vi "Multiple AOIs.vi"(4 "White level":dbl=255.0 format="%.2f", 5 "Black level":dbl format="%.2f", 6 "First (or only) image (red)":T2, 8 "error in":errorcluster, 9 "Second image (green)":T2, 11 "Image Type":u32(ring) items=["8 bits", "16 bits", "Float", "Complex", "RGB", "HSL"]) -> (0 "error out":errorcluster)   [LabVIEW 2011]
doc: "Use to designate multiple areas of interest (AOIs) in the image"
uses:
  <vilib>/vision/Image Controls.llb/IMAQ Image.ctl
  AOI List Globals.vi
  <vilib>/vision/NI_Vision_Development_Module.lvlib
  <vilib>/Utility/NIReport.llb/NI_ReportGenerationCore.lvlib
  <vilib>/Analysis/NI_AALBase.lvlib
panel:
  in  "Case Constant\n(See Context Help)":bool
  in  "Printer":u16(ring) items=["QBIO lab Lexmark C532 PS3", "Microsoft XPS Document Writer", "Microsoft Office Document Image Writer", "Lab Zippy  (jg-zippy.kosow.brandeis.edu)", "Lab hp color LaserJet 2550 PS", "Journal Note Writer", "HP Universal Printing PS", "HP Universal Printing PCL 6", "Home HP LaserJet 4L", "Fax", "Adobe PDF", "\\\\BASEMENT\\Home EPSON Stylus Photo 1400 Series", "\\\\jg-x\\Jeff's office EPSON Stylus CX7400 Series 2"]
  in  "Print AOIs":bool
  in  "Resize all AOIs":bool
  in  "Read AOI list from file":bool
  in  "Save AOI list to file":bool
  in  "Y":u16(slide)=20 caption="Fixed AOI Y size" max=480 scale=0.0..50.0
  in  "X":u16(slide)=20 caption="Fixed AOI X size" max=640 scale=0.0..50.0
  in  "Delete all AOIs":bool
  in  "Mouse Operation to perform":T1(ring)
  in  "Exit":bool
  # "Ordinarily not for interactive use:"
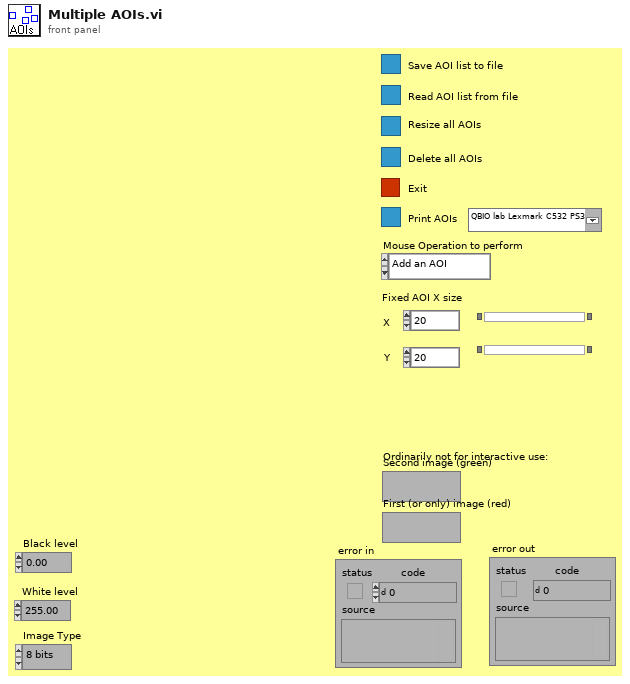
[diagram p1: front panel]
types:
  T1 = enum16{"Add an AOI", "Resize an AOI", "Delete an AOI"}
  T2 = typedef "IMAQ Image.ctl" = refnum<image>
  T3 = enum32{"8 bits", "16 bits", "Float", "Complex", "RGB Chunky", "Compressed"}
  T4 = enum32{"No Selection", "Point", "Line", "Rectangle", "Oval", "Polygon", "Free", "Unused1", "Zoom", "Unused2", "Broken Line", "Free Hand Line"}
  T5 = enum32{"No Selection", "Point", "Line", "Rectangle", "Oval", "Polygon", "Free", "Unused1", "Zoom", "Unused2", "Broken Line", "Free Hand Line"}[]
  T6 = enum32{"No  event", "Click event", "Draw event", "Move event", "Size event", "Scroll event", "Activate event", "Close event", "Reserved"}[]
  T7 = cluster{"AOI List[0]":u16, "AOI List[1]":u16, "AOI List[2]":u16, "AOI List[3]":u16}
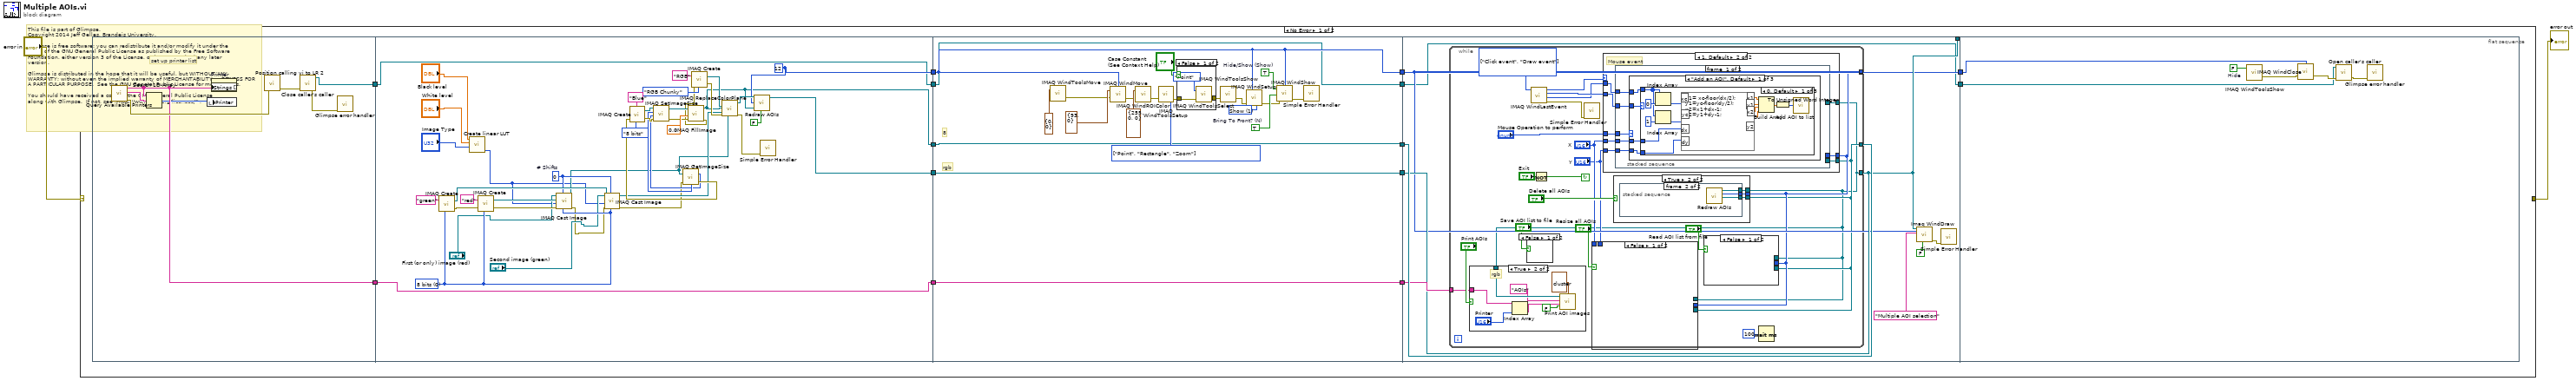
[diagram p0: block diagram]
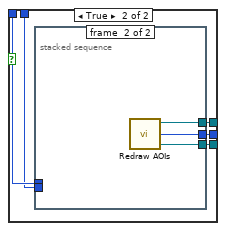
[diagram p4: hidden frame]
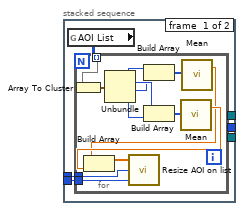
[diagram p5: hidden frame]
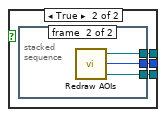
[diagram p6: hidden frame]
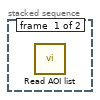
[diagram p7: hidden frame]
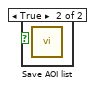
[diagram p8: hidden frame]
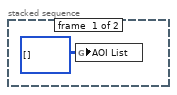
[diagram p10: hidden frame]
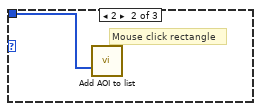
[diagram p12: hidden frame]
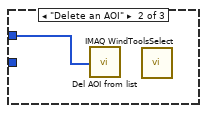
[diagram p14: hidden frame]
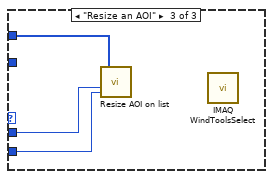
[diagram p15: hidden frame]
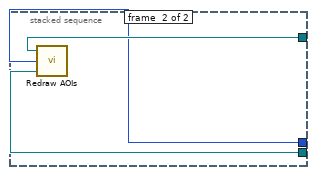
[diagram p16: hidden frame]
diagram:
  # "This file is part of Glimpse. \nCopyright 2014 Jeff Gelles, Brandeis University.    \n\nGlimpse is free software: you can redistribute it and/or modify it under the \nterms of the GNU General Public License as published by the Free Software \nFoundation, either version 3 of the License, or (at your option) any later \nversion.\n\nGlimpse is distributed in the hope that it will be useful, but WITHOUT ANY \nWARRANTY; without even the implied warranty of MERCHANTABILITY or FITNESS FOR \nA PARTICULAR PURPOSE.  See the GNU General Public License for more details.\n\nYou should have received a copy of the GNU General Public License\nalong with Glimpse.  If not, see <http://www.gnu.org/licenses/>."
  n1 = case shown="No Error" "error in" {
    selector: "error in" -> [_ w206]
    tunnel: [_ w206] -> w1
    frame No Error {
      n2 = flat-sequence {
        tunnel: [w22] -> w16
        tunnel: [w19] -> w15
        tunnel: [w50] -> w14
        tunnel: [w52] -> w13
        tunnel: [w38] -> w12
        tunnel: w16 -> [w25]
        tunnel: [w25] -> w11
        tunnel: w15 -> [w24]
        tunnel: [w24] -> w10
        tunnel: w14 -> [w69]
        tunnel: [w69] -> w9
        tunnel: w13 -> [w68]
        tunnel: [w68] -> w8
        tunnel: w12 -> [w67]
        tunnel: [w67] -> w7
        tunnel: w11 -> [w66]
        tunnel: [w66] -> w6
        tunnel: w10 -> [w65]
        tunnel: [w65] -> w5
        tunnel: [w95] -> _
        tunnel: w9 -> [w91]
        tunnel: [w91] -> w4
        tunnel: w8 -> [w95]
        tunnel: w7 -> [w97]
        tunnel: w6 -> [w90]
        tunnel: [w90] -> w3
        tunnel: w5 -> [w96]
        tunnel: w4 -> [w204]
        tunnel: w3 -> [w200]
        frame #0 {
          # "set up printer list"
          n3 = call <vilib>:"Query Available Printers.vi"() -> ("error out"=w20:errorcluster, "default printer"=w18:string, "system configured printers"=w19:string[])  [unwired: 1 in, 8 out]
          n4 = Search 1D Array(1D array=w19, element=w18) -> (index of element=w17:i32)  [unwired: 1 out]
          n5 = local write "Printer"(w17) -> ()
          n6 = property on="Printer" class="Ring (strict)"("Strings []"=w19) -> ()  [unwired: 2 in, 2 out]
          n7 = call "Position calling vi to LR 2.vi"("error in (no error)"=w20) -> ("error out"=w23:errorcluster)  [unwired: 1 in, 3 out]
          n8 = call "Close caller's caller.vi"("error in (no error)"=w23) -> ("error out"=w21:errorcluster, "vi reference"=w22:refnum<vi>)  [unwired: 6 out]
          n9 = call "Glimpse error handler.vi"("error in"=w21) -> ()  [unwired: 1 in, 6 out]
        }
        frame #1 {
          w39 = 0  # # Shifts
          w44 = u32 0 items=["8 bits", "16 bits", "Float", "Complex", "RGB", "HSL"] ("Image Type")
          w50 = 12 ("Window Number (0...15)")
          n10 = call "IMAQ Create"("Image Name"="green", "Image Type"=w44) -> ("New Image"=w42:T2, "error out"=w45:errorcluster)  [unwired: 2 in, 1 out]
          n11 = call "Create linear LUT.vi"("Input Image Type"="Image Type", "White Value"="White level", "Black Value"="Black level") -> ("LUT (U8) Out"=w28:u8[])  [unwired: 1 in, 5 out]
          n12 = call "IMAQ Create"("Image Name"="red", "Image Type"=w44, "error in (no error)"=w45) -> ("New Image"=w43:T2, "error out"=w31:errorcluster)  [unwired: 1 in, 1 out]
          n13 = call "IMAQ Cast Image"("Image Type"=w44, "# Shifts"=w39, "error in (no error)"=w31, "Lookup Table"=w28, "Image Dst"=w43, "Image Src"="First (or only) image (red)") -> ("error out"=w27:errorcluster, "Image Dst Out"=w37:T2)  [unwired: 4 out]
          n14 = call "IMAQ Cast Image"("Image Type"=w44, "# Shifts"=w39, "error in (no error)"=w27, "Lookup Table"=w28, "Image Dst"=w42, "Image Src"="Second image (green)") -> ("error out"=w46:errorcluster, "Image Dst Out"=w47:T2)  [unwired: 4 out]
          n15 = call "IMAQ GetImageSize"("Image"=w37, "error in (no error)"=w46) -> ("Y Resolution"=w48:i32, "X Resolution"=w49:i32, "error out"=w53:errorcluster)  [unwired: 2 out]
          n16 = call "IMAQ Create"("Image Name"="Blue", "Image Type"=T3."8 bits", "error in (no error)"=w53) -> ("New Image"=w57:T2, "error out"=w56:errorcluster)  [unwired: 1 in, 1 out]
          n17 = call "IMAQ SetImageSize"("error in (no error)"=w56, "Y Resolution"=w48, "X Resolution"=w49, "Image"=w57) -> ("error out"=w54:errorcluster, "Image Out"=w55:T2)  [unwired: 1 out]
          n18 = call "IMAQ FillImage"("error in (no error)"=w54, "Pixel Value (U8, U16, I16, Float)"=sgl 0.0 ("Pixel Value (U8, I16, Float)"), "Image"=w55) -> ("error out"=w33:errorcluster, "Image Out"=w38:T2)  [unwired: 4 in, 3 out]
          n19 = call "IMAQ Create"("Image Name"="RGB", "Image Type"=T3."RGB Chunky", "error in (no error)"=w33) -> ("New Image"=w62:T2, "error out"=w61:errorcluster)  [unwired: 1 in, 1 out]
          n20 = call "IMAQ ReplaceColorPlane"("Image Dst"=w62, "Red or Hue Plane"=w38, "Green or Sat Plane"=w47, "error in (no error)"=w61, "Blue or Luma or Val or Inten Plane"=w37) -> ("Image Dst Out"=w51:T2, "error out"=w32:errorcluster)  [unwired: 2 in, 7 out]
          n21 = call "Redraw AOIs.vi"("Resize to Image Size?"=FALSE, "Image Src (Red Plane)"=w38, "Window Number (0...15)"=w50, "Image Src (RGB)"=w51) -> ("Image Dst Out (RGB)"=w52:T2)  [unwired: 1 out]
          n22 = call <vilib>:"Simple Error Handler.vi"("error in (no error)"=w32) -> ()  [unwired: 1 in, 8 out]
        }
        frame #2 {
          w70 = 1 items=["Hide", "Show", "No change"] ("Scrollbars (No change)")
          w77 = TRUE  # Bring To Front? (N)
          w78 = TRUE  # Hide/Show (Show)
          w83 = T5 [enum."Point", enum."Rectangle", enum."Zoom"] items=["No Selection", "Point", "Line", "Rectangle", "Oval", "Polygon", "Free", "Unused1", "Zoom", "Unused2", "Broken Line", "Free Hand Line"] ("Tools")
          # "rgb"
          # "8"
          n23 = call "IMAQ WindToolsMove"("Coordinates"=cluster{"X Position":i32, "Y Position":i32} {"X Position"=0, "Y Position"=0}) -> ("error out"=w73:errorcluster)  [unwired: 2 in, 3 out]
          n24 = call "IMAQ WindMove"("Window Number (0...15)"=w69, "Coordinates (screen)"=cluster{"X Position":i32, "Y Position":i32} {"X Position"=93, "Y Position"=0}, "error in (no error)"=w73) -> ("error out"=w72:errorcluster)  [unwired: 1 in, 2 out]
          n25 = call "IMAQ WindROIColor"("Color of ROI (white)"=cluster{"Red":u8, "Green":u8, "Blue":u8} {"Red"=255, "Green"=0, "Blue"=0}, "error in (no error)"=w72) -> ("error out"=w84:errorcluster)  [unwired: 4 out]
          n26 = call "IMAQ WindToolsSetup"("Tools"=w83, "error in (no error)"=w84) -> ("error out"=w82:errorcluster)  [unwired: 2 in, 2 out]
          n27 = case shown="False" "Case Constant\n(See Context Help)" {
            tunnel: w82 -> [w87 w89]
            tunnel: [w86 w89] -> w81
            frame False {
              n28 = call "IMAQ WindToolsSelect"("Tool (Point)"=T4."Point", "error in (no error)"=w87) -> ("error out"=w86:errorcluster)  [unwired: 2 in, 2 out]
            }
            frame True {
            }
          }
          n29 = call "IMAQ WindToolsShow"("error in (no error)"=w81) -> ("error out"=w80:errorcluster)  [unwired: 2 in, 3 out]
          n30 = call "IMAQ WindSetup"("Scrollbars (No change)"=w70, "Window Number (0...15)"=w69, "error in (no error)"=w80) -> ("error out"=w71:errorcluster)  [unwired: 4 in, 4 out]
          n31 = call "IMAQ WindShow"("error in (no error)"=w71, "Bring To Front? (N)"=w77, "Hide/Show (Show)"=w78, "Window Number (0...15)"=w69) -> ("error out"=w79:errorcluster)  [unwired: 1 in, 3 out]
          n32 = call <vilib>:"Simple Error Handler.vi"("error in (no error)"=w79) -> ()  [unwired: 1 in, 8 out]
        }
        frame #3 {
          n33 = while {
            tunnel: w95 -> [w99]
            tunnel: w97 -> [w103]
            tunnel: w91 -> [w104]
            tunnel: w91 -> [_]
            tunnel: w96 -> [w98]
            stop <- w116 continue-if-true
            w115 = T6 [enum."Click event", enum."Draw event"] items=["No  event", "Click event", "Draw event", "Move event", "Size event", "Scroll event", "Activate event", "Close event", "Reserved"] ("Events list (all)")
            n34 = case shown="True" "Print AOIs" {
              tunnel: w99 -> [_ w124]
              tunnel: w98 -> [_ w121]
              frame False {
              }
              frame True {
                # "rgb"
                n35 = Index Array(array=w121, index="Printer") -> (element=w123:string)
                n36 = call "Print AOI images.vi"("Black/White Levels"=cluster{ext, ext} {0.0, 255.0}, "AOI Overlay?"=FALSE, "printer name (default)"=w123, "Printout title"="AOIs", "Image In"=w124) -> ()  [unwired: 1 in, 5 out]
              }
            }
            n37 = case shown="False" "Save AOI list to file" {
              frame False {
              }
              frame True {
                n38 = call "Save AOI list.vi"() -> ()  [unwired: 1 out]
              }
            }
            n39 = call "IMAQ WindLastEvent"("Events list (all)"=w115) -> ("error out"=w101:errorcluster, "Coordinates"=w111:i32[], "Tool"=w112:i32, "Event"=w114:i32)  [unwired: 1 in, 6 out]
            n40 = Not(x="Exit") -> (.not. x?=w116:bool)
            n41 = call <vilib>:"Simple Error Handler.vi"("error in (no error)"=w101) -> ()  [unwired: 1 in, 8 out]
            n42 = case shown="False" "Resize all AOIs" {
              tunnel: "X" -> [_ w129]
              tunnel: "Y" -> [_ w128]
              tunnel: w99 -> [_ w127]
              tunnel: w104 -> [_ w126]
              tunnel: w103 -> [_ w125]
              frame False {
              }
              frame True {
                n43 = stacked-sequence {
                  tunnel: w129 -> [w132 _]
                  tunnel: w128 -> [w131 _]
                  tunnel: w127 -> [_ w148]
                  tunnel: w126 -> [_ w147]
                  tunnel: w125 -> [_ w146]
                  frame #0 {
                    n44 = global read "AOI List Globals.vi" "AOI List"() -> (w130:u16[][])
                    n45 = for {
                      tunnel: w132 -> [w145]
                      tunnel: w131 -> [w144]
                      tunnel: w130 -> [w142] mode=indexing
                      n46 = Array To Cluster(array=w142) -> (cluster=w141:T7)
                      n47 = Unbundle(w141) -> ("AOI List[0]"=w140:u16, "AOI List[1]"=w139:u16, "AOI List[2]"=w138:u16, "AOI List[3]"=w137:u16)
                      n48 = Build Array(w140, w138) -> (w136:u16[])
                      n49 = Build Array(w139, w137) -> (w135:u16[])
                      n50 = call <vilib>:"Mean.vi"("X"=w135) -> ("mean"=w134:dbl)  [unwired: 1 out]
                      n51 = call <vilib>:"Mean.vi"("X"=w136) -> ("mean"=w133:dbl)  [unwired: 1 out]
                      n52 = Build Array(w133, w134) -> (w143:dbl[])
                      n53 = call "Resize AOI on list.vi"("New y dimension"=w144, "New x dimension"=w145, "Coordinates of  AOI to resize"=w143) -> ()  [unwired: 2 out]
                    }
                  }
                  frame #1 {
                    n54 = call "Redraw AOIs.vi"("Image Src (Red Plane)"=w146, "Window Number (0...15)"=w147, "Image Src (RGB)"=w148) -> ()  [unwired: 1 in, 2 out]
                  }
                }
              }
            }
            n55 = case shown="1, Default" w114 {
              tunnel: "Mouse Operation to perform" -> [_ w169]
              tunnel: w112 -> [_ w168]
              tunnel: w111 -> [_ w167]
              tunnel: w104 -> [_ w166]
              tunnel: w103 -> [_ w165]
              tunnel: w99 -> [_ w164]
              tunnel: "X" -> [_ w163]
              tunnel: "Y" -> [_ w162]
              frame 0 {
                # "No mouse event"
              }
              frame 1, Default {
                # "Mouse event"
                n56 = stacked-sequence {
                  tunnel: w169 -> [w174 _]
                  tunnel: w168 -> [w173 _]
                  tunnel: w167 -> [w172 _]
                  tunnel: w166 -> [_ w198]
                  tunnel: w165 -> [_ w197]
                  tunnel: w164 -> [_ w199]
                  tunnel: w163 -> [w171 _]
                  tunnel: w162 -> [w170 _]
                  frame #0 {
                    n57 = case shown="\"Add an AOI\", Default" w174 {
                      tunnel: w173 -> [w178 _ _]
                      tunnel: w172 -> [w177 w193 w194]
                      tunnel: w171 -> [w176 _ w196]
                      tunnel: w170 -> [w175 _ w195]
                      frame "Add an AOI", Default {
                        n58 = case shown="0, Default" w178 {
                          tunnel: w177 -> [w189 w192 _]
                          tunnel: w176 -> [w182 _ _]
                          tunnel: w175 -> [w181 _ _]
                          frame 0, Default {
                            # "Mouse click point"
                            n59 = Index Array(array=w189, index=0) -> (element=w188:i32)
                            n60 = Index Array(array=w189, index=1) -> (element=w187:i32)
                            n61 = formula code="x1= xc-floor(dx/2);\ny1=yc-floor(dy/2);\nx2=x1+dx-1;\ny2=y1+dy-1;"("xc"=w188, "yc"=w187, "dx"=w182, "dy"=w181) -> ("x1"=w185:dbl, "y1"=w186:dbl, "x2"=w184:dbl, "y2"=w183:dbl)
                            n62 = Build Array(w185, w186, w184, w183) -> (w179:dbl[])
                            n63 = To Unsigned Word Integer(number=w179) -> (unsigned 16bit integer=w180:u16[])
                            n64 = call "Add AOI to list.vi"("AOI to add"=w180) -> ()  [unwired: 1 out]
                          }
                          frame 2 {
                            # "Mouse click rectangle"
                            n65 = call "Add AOI to list.vi"("AOI to add"=w192) -> ()  [unwired: 1 out]
                          }
                          frame 8 {
                            # "zoom -- no action"
                          }
                        }
                      }
                      frame "Delete an AOI" {
                        n66 = call "Del AOI from list.vi"("Coordinates of  AOI to delete"=w193) -> ()  [unwired: 1 out]
                        n67 = call "IMAQ WindToolsSelect"() -> ()  [unwired: 4 in, 3 out]
                      }
                      frame "Resize an AOI" {
                        n68 = call "Resize AOI on list.vi"("New y dimension"=w195, "New x dimension"=w196, "Coordinates of  AOI to resize"=w194) -> ()  [unwired: 2 out]
                        n69 = call "IMAQ WindToolsSelect"() -> ()  [unwired: 4 in, 3 out]
                      }
                    }
                  }
                  frame #1 {
                    n70 = call "Redraw AOIs.vi"("Image Src (Red Plane)"=w197, "Window Number (0...15)"=w198, "Image Src (RGB)"=w199) -> ()  [unwired: 1 in, 2 out]
                  }
                }
              }
            }
            n71 = case shown="True" "Delete all AOIs" {
              tunnel: w104 -> [_ w157]
              tunnel: w103 -> [_ w156]
              tunnel: w99 -> [_ w155]
              frame False {
              }
              frame True {
                n72 = stacked-sequence {
                  tunnel: w157 -> [_ w160]
                  tunnel: w156 -> [_ w159]
                  tunnel: w155 -> [_ w161]
                  frame #0 {
                    n73 = global write "AOI List Globals.vi" "AOI List"(i32[][] []) -> ()
                  }
                  frame #1 {
                    n74 = call "Redraw AOIs.vi"("Image Src (Red Plane)"=w159, "Window Number (0...15)"=w160, "Image Src (RGB)"=w161) -> ()  [unwired: 1 in, 2 out]
                  }
                }
              }
            }
            n75 = case shown="False" "Read AOI list from file" {
              tunnel: w99 -> [_ w151]
              tunnel: w104 -> [_ w150]
              tunnel: w103 -> [_ w149]
              frame False {
              }
              frame True {
                n76 = stacked-sequence {
                  tunnel: w151 -> [_ w154]
                  tunnel: w150 -> [_ w153]
                  tunnel: w149 -> [_ w152]
                  frame #0 {
                    n77 = call "Read AOI list.vi"() -> ()  [unwired: 2 out]
                  }
                  frame #1 {
                    n78 = call "Redraw AOIs.vi"("Image Src (Red Plane)"=w152, "Window Number (0...15)"=w153, "Image Src (RGB)"=w154) -> ()  [unwired: 1 in, 2 out]
                  }
                }
              }
            }
            n79 = Wait (ms)(milliseconds to wait=u32 100) -> ()  [unwired: 1 out]
          }
          n80 = call "Imaq WindDraw"("Resize to Image Size? (Y)"=FALSE, "Window Number (0...15)"=w91, "Title"="Multiple AOI selection", "Image"=w95) -> ("error out"=w93:errorcluster)  [unwired: 2 in, 5 out]
          n81 = call <vilib>:"Simple Error Handler.vi"("error in (no error)"=w93) -> ()  [unwired: 1 in, 8 out]
        }
        frame #4 {
          w205 = FALSE  # Hide
          n82 = call "IMAQ WindToolsShow"("Hide/Show (Show)"=w205) -> ("error out"=w203:errorcluster)  [unwired: 2 in, 3 out]
          n83 = call "IMAQ WindClose"("Window Number (0...15)"=w204, "error in (no error)"=w203) -> ("error out"=w202:errorcluster)  [unwired: 1 in, 3 out]
          n84 = call "Open caller's caller.vi"("error in (no error)"=w202, "vi reference"=w200) -> ("error out"=w201:errorcluster)  [unwired: 6 out]
          n85 = call "Glimpse error handler.vi"("error in"=w201) -> ()  [unwired: 1 in, 6 out]
        }
      }
    }
    frame Error {
    }
  }
  "error out" <- w1
